vi "CMD_SERIALECHO.vi"(6 "Gantry in":refnum<class "Gantry.lvclass">, 7 "Console Log in":refnum<class "Console Log.lvclass">, 8 "error in (no error)":errorcluster, 10 "Arguments":string[](array[string]), 11 "gScript Interpreter in":refnum<class "gScript Interpreter.lvclass">) -> (0 "error out":errorcluster, 3 "gScript Interpreter out":refnum<class "gScript Interpreter.lvclass">, 4 "Gantry out":refnum<class "Gantry.lvclass">, 5 "Console Log out":refnum<class "Console Log.lvclass">)   [LabVIEW 2024, in "gScript Interpreter.lvclass"]
uses:
  gScript Interpreter.lvclass
  Shared Components/Gantry Class/Gantry.lvclass
  Application Utilities/Console Log/Console Log.lvclass
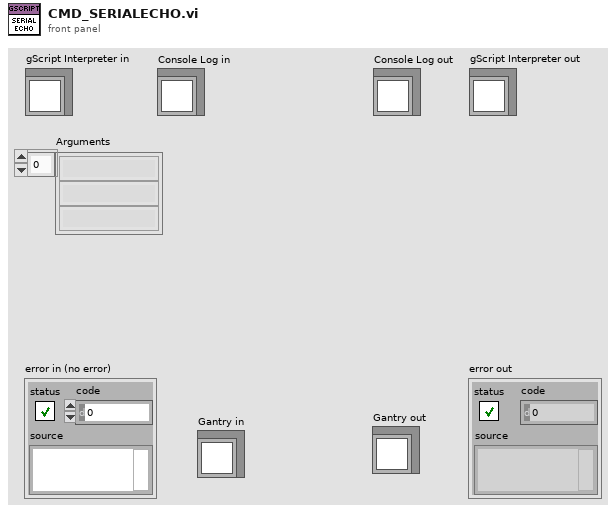
[diagram p1: front panel]
types:
  T1 = typedef "Memory Cell.ctl" = cluster{"type":T2, "x":dbl, "y":dbl, "z":dbl, "w":dbl}
  T2 = typedef "Memory Cell Type Enum.ctl" = enum16{"integer", "float", "vector", "rotation"}
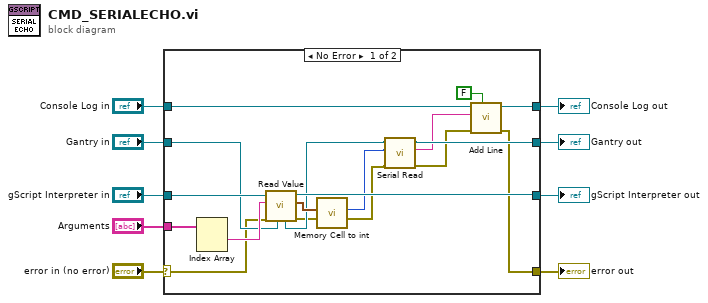
[diagram p0: block diagram]
diagram:
  n1 = case shown="No Error" "error in (no error)" {
    selector: "error in (no error)" -> [w20 w30]
    tunnel: [w10 w30] -> w8
    tunnel: [w23 w29] -> w6
    tunnel: "gScript Interpreter in" -> [w22 w29]
    tunnel: "Arguments" -> [w26 _]
    tunnel: "Gantry in" -> [w21 w28]
    tunnel: [w18 w28] -> w3
    tunnel: "Console Log in" -> [w15 w27]
    tunnel: [w14 w27] -> w1
    frame No Error {
      n2 = Index Array(array=w26) -> (element #1=w25:string)  [unwired: 2 in, 1 out]
      n3 = call-dynamic "Read Value.vi"("Gantry in"=w21, "error in (no error)"=w20, "String in"=w25, "gScript Interpreter in"=w22) -> ("error out"=w17:errorcluster, "Memory Cell"=w24:T1, "gScript Interpreter out"=w23:refnum<class "gScript Interpreter.lvclass">, "Gantry out"=w19:refnum<class "Gantry.lvclass">)  [unwired: 4 in]
      n4 = call "Memory Cell to int.vi"("Memory Cell"=w24) -> ("Int out"=w16:i32)  [unwired: 10 in]
      n5 = call "Serial Read.vi"("error in (no error)"=w17, "Connection ID"=w16, "Gantry in"=w19) -> ("error out"=w11:errorcluster, "read buffer"=w12:string, "Gantry out"=w18:refnum<class "Gantry.lvclass">)  [unwired: 6 in]
      n6 = call "Add Line.vi"("Timestamp"=FALSE, "error in"=w11, "String"=w12, "Console Log in"=w15) -> ("error out"=w10:errorcluster, "Console Log out"=w14:refnum<class "Console Log.lvclass">)  [unwired: 6 in]
    }
    frame Error {
    }
  }
  "error out" <- w8
  "gScript Interpreter out" <- w6
  "Gantry out" <- w3
  "Console Log out" <- w1
